vi "Status to Cluster.vi"(11 "Status":string) -> (3 "Status Cluster":T1)   [LabVIEW 2021, in "Keysight U1282A.lvlib"]
doc: "Este VI regresa la interpretación del status del instrumento (cadena de carácteres) en forma de un cluster de indicadores."
uses:
  Keysight U1282A.lvlib
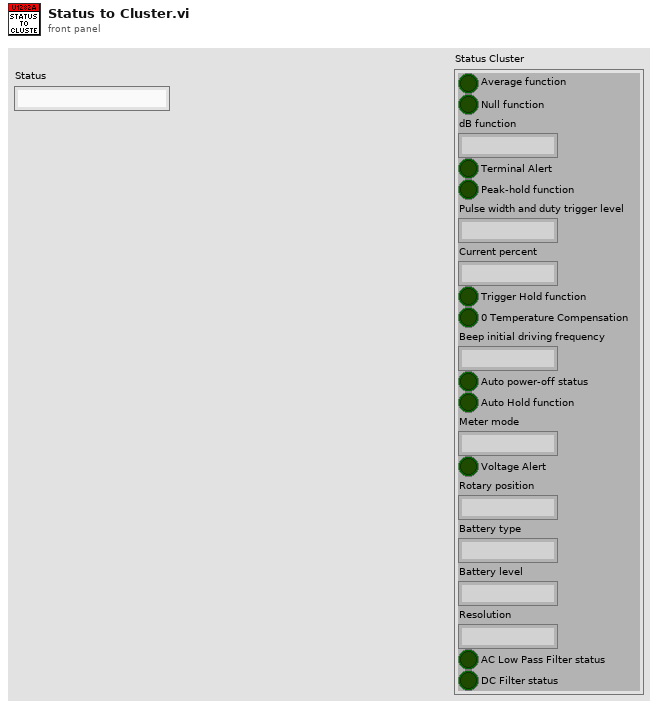
[diagram p1: front panel]
types:
  T1 = cluster{"Average function":bool, "Null function":bool, "dB function":string, "Terminal Alert":bool, "Peak-hold function":bool, "Pulse width and duty trigger level":string, "Current percent ":string, "Trigger Hold function":bool, "0 Temperature Compensation":bool, "Beep initial driving frequency":string, "Auto power-off status":bool, "Auto Hold function":bool, "Meter mode":string, "Voltage Alert":bool, "Rotary position":string, "Battery type":string, "Battery level":string, "Resolution":string, "AC Low Pass Filter status":bool, "DC Filter status":bool}
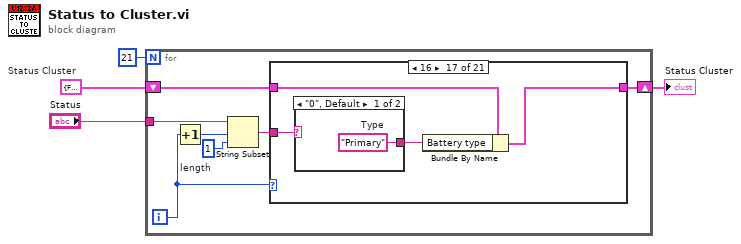
[diagram p0: block diagram]
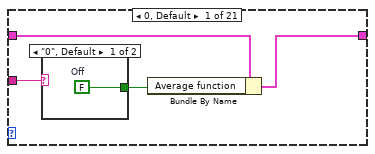
[diagram p2: hidden frame]
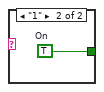
[diagram p3: hidden frame]
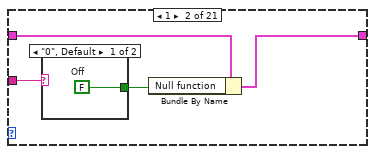
[diagram p4: hidden frame]
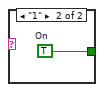
[diagram p5: hidden frame]
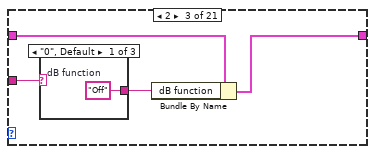
[diagram p6: hidden frame]
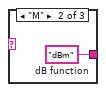
[diagram p7: hidden frame]
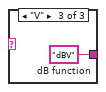
[diagram p8: hidden frame]
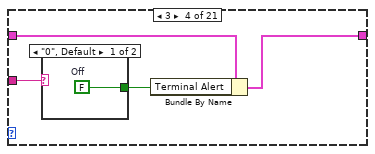
[diagram p9: hidden frame]
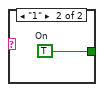
[diagram p10: hidden frame]
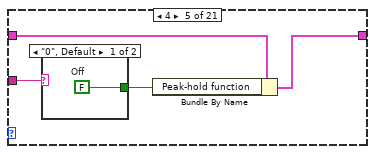
[diagram p11: hidden frame]
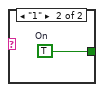
[diagram p12: hidden frame]
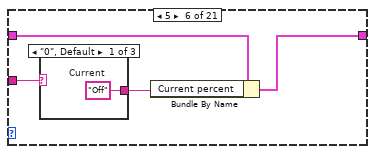
[diagram p13: hidden frame]
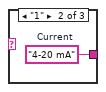
[diagram p14: hidden frame]
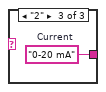
[diagram p15: hidden frame]
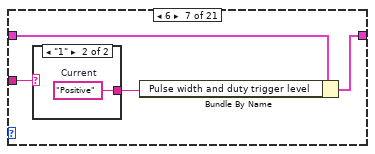
[diagram p16: hidden frame]
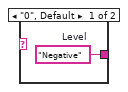
[diagram p17: hidden frame]
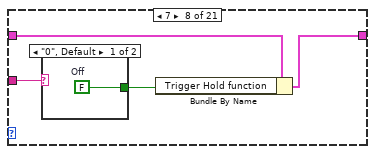
[diagram p18: hidden frame]
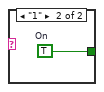
[diagram p19: hidden frame]
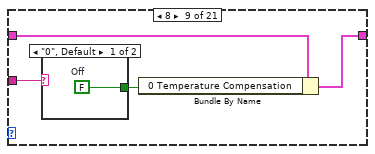
[diagram p20: hidden frame]
diagram:
  w1 = T1 {"Average function"=FALSE, "Null function"=FALSE, "dB function"="", "Terminal Alert"=FALSE, "Peak-hold function"=FALSE, "Pulse width and duty trigger level"="", "Current percent "="", "Trigger Hold function"=FALSE, "0 Temperature Compensation"=FALSE, "Beep initial driving frequency"="", "Auto power-off status"=FALSE, "Auto Hold function"=FALSE, "Meter mode"="", "Voltage Alert"=FALSE, "Rotary position"="", "Battery type"="", "Battery level"="", "Resolution"="", "AC Low Pass Filter status"=FALSE, "DC Filter status"=FALSE}  # Status Cluster
  n1 = for {
    N: 21 -> [_]
    tunnel: "Status" -> [w11]
    shift-right: [w8] -> w3
    shift-left: w1 -> [w9]
    i -> [w6]
    w10 = 1  # length
    n2 = Increment(x=w6) -> (x+1=w5:i32)
    n3 = String Subset(string=w11, offset (0)=w5, length (rest)=w10) -> (substring=w7:string)
    n4 = case shown="16" w6 {
      tunnel: w9 -> [w12 w18 w24 w34 w37 w43 w50 w56 w62 w68 w86 w95 w101 w107 w110 w111 w126 w134 w137 w143 w150]
      tunnel: [w13 w21 w27 w33 w40 w46 w53 w59 w65 w71 w89 w94 w100 w106 w110 w114 w125 w133 w140 w146 w149] -> w8
      tunnel: w7 -> [w15 w20 w26 w32 w39 w45 w52 w58 w64 w70 w88 w93 w99 w105 _ w113 w128 w132 w139 w145 w152]
      frame 0, Default {
        n5 = case shown="\"0\", Default" w15 {
          tunnel: [w16 w17] -> w14
          frame "0", Default {
            w16 = FALSE  # Off
          }
          frame "1" {
            w17 = TRUE  # On
          }
        }
        n6 = Bundle By Name(cluster=w12, "Average function"=w14) -> (w13:T1)
      }
      frame 1 {
        n7 = case shown="\"0\", Default" w20 {
          tunnel: [w22 w23] -> w19
          frame "0", Default {
            w22 = FALSE  # Off
          }
          frame "1" {
            w23 = TRUE  # On
          }
        }
        n8 = Bundle By Name(cluster=w18, "Null function"=w19) -> (w21:T1)
      }
      frame 2 {
        n9 = case shown="\"0\", Default" w26 {
          tunnel: [w28 w29 w30] -> w25
          frame "0", Default {
            w28 = "Off"  # dB function
          }
          frame "M" {
            w29 = "dBm"  # dB function
          }
          frame "V" {
            w30 = "dBV"  # dB function
          }
        }
        n10 = Bundle By Name(cluster=w24, "dB function"=w25) -> (w27:T1)
      }
      frame 3 {
        n11 = case shown="\"0\", Default" w32 {
          tunnel: [w35 w36] -> w31
          frame "0", Default {
            w35 = FALSE  # Off
          }
          frame "1" {
            w36 = TRUE  # On
          }
        }
        n12 = Bundle By Name(cluster=w34, "Terminal Alert"=w31) -> (w33:T1)
      }
      frame 4 {
        n13 = case shown="\"0\", Default" w39 {
          tunnel: [w41 w42] -> w38
          frame "0", Default {
            w41 = FALSE  # Off
          }
          frame "1" {
            w42 = TRUE  # On
          }
        }
        n14 = Bundle By Name(cluster=w37, "Peak-hold function"=w38) -> (w40:T1)
      }
      frame 5 {
        n15 = case shown="\"0\", Default" w45 {
          tunnel: [w47 w48 w49] -> w44
          frame "0", Default {
            w47 = "Off"  # Current
          }
          frame "1" {
            w48 = "4-20 mA"  # Current
          }
          frame "2" {
            w49 = "0-20 mA"  # Current
          }
        }
        n16 = Bundle By Name(cluster=w43, "Current percent"=w44) -> (w46:T1)
      }
      frame 6 {
        n17 = case shown="\"1\"" w52 {
          tunnel: [w54 w55] -> w51
          frame "0", Default {
            w54 = "Negative"  # Level
          }
          frame "1" {
            w55 = "Positive"  # Current
          }
        }
        n18 = Bundle By Name(cluster=w50, "Pulse width and duty trigger level"=w51) -> (w53:T1)
      }
      frame 7 {
        n19 = case shown="\"0\", Default" w58 {
          tunnel: [w60 w61] -> w57
          frame "0", Default {
            w60 = FALSE  # Off
          }
          frame "1" {
            w61 = TRUE  # On
          }
        }
        n20 = Bundle By Name(cluster=w56, "Trigger Hold function"=w57) -> (w59:T1)
      }
      frame 8 {
        n21 = case shown="\"0\", Default" w64 {
          tunnel: [w66 w67] -> w63
          frame "0", Default {
            w66 = FALSE  # Off
          }
          frame "1" {
            w67 = TRUE  # On
          }
        }
        n22 = Bundle By Name(cluster=w62, "0 Temperature Compensation"=w63) -> (w65:T1)
      }
      frame 9 {
        n23 = case shown="\"9\"" w70 {
          tunnel: [w72 w73 w74 w75 w76 w77 w78 w79 w80 w81 w82 w83 w84 w85] -> w69
          frame "0", Default {
            w72 = "Off"  # Frequency
          }
          frame "1" {
            w73 = "3200 Hz"  # Frequency
          }
          frame "2" {
            w74 = "3268 Hz"  # Frequency
          }
          frame "3" {
            w75 = "3339 Hz"  # Frequency
          }
          frame "4" {
            w76 = "3413 Hz"  # Frequency
          }
          frame "5" {
            w77 = "3491 Hz"  # Frequency
          }
          frame "6" {
            w78 = "3572 Hz"  # Frequency
          }
          frame "7" {
            w79 = "3657 Hz"  # Frequency
          }
          frame "8" {
            w80 = "3746 Hz"  # Frequency
          }
          frame "9" {
            w81 = "3840 Hz"  # Frequency
          }
          frame "A" {
            w82 = "3938 Hz"  # Frequency
          }
          frame "B" {
            w83 = "4042 Hz"  # Frequency
          }
          frame "C" {
            w84 = "4151 Hz"  # Frequency
          }
          frame "D" {
            w85 = "4267 Hz"  # Frequency
          }
        }
        n24 = Bundle By Name(cluster=w68, "Beep initial driving frequency"=w69) -> (w71:T1)
      }
      frame 10 {
        n25 = case shown="\"1\"" w88 {
          tunnel: [w90 w91] -> w87
          frame "0", Default {
            w90 = FALSE  # Off
          }
          frame "1" {
            w91 = TRUE  # On
          }
        }
        n26 = Bundle By Name(cluster=w86, "Auto power-off status"=w87) -> (w89:T1)
      }
      frame 11 {
        n27 = case shown="\"0\", Default" w93 {
          tunnel: [w96 w97] -> w92
          frame "0", Default {
            w96 = FALSE  # Off
          }
          frame "1" {
            w97 = TRUE  # On
          }
        }
        n28 = Bundle By Name(cluster=w95, "Auto Hold function"=w92) -> (w94:T1)
      }
      frame 12 {
        n29 = case shown="\"L\", Default" w99 {
          tunnel: [w102 w103] -> w98
          frame "L", Default {
            w102 = "Normal"  # Mode
          }
          frame "C" {
            w103 = "Calibraition"  # Mode
          }
        }
        n30 = Bundle By Name(cluster=w101, "Meter mode"=w98) -> (w100:T1)
      }
      frame 13 {
        n31 = case shown="\"0\", Default" w105 {
          tunnel: [w108 w109] -> w104
          frame "0", Default {
            w108 = FALSE  # Off
          }
          frame "1" {
            w109 = TRUE  # On
          }
        }
        n32 = Bundle By Name(cluster=w107, "Voltage Alert"=w104) -> (w106:T1)
      }
      frame 14 {
      }
      frame 15 {
        n33 = case shown="\"2\"" w113 {
          tunnel: [w115 w116 w117 w118 w119 w120 w121 w122 w123 w124] -> w112
          frame "0", Default {
            w115 = "ACV"  # Measurement
          }
          frame "1" {
            w116 = "ACmV"  # Measurement
          }
          frame "2" {
            w117 = "ACDCV"  # Measurement
          }
          frame "3" {
            w118 = "ACDCmV"  # Measurement
          }
          frame "4" {
            w119 = "Ohm/nS"  # Measurement
          }
          frame "5" {
            w120 = "Diode"  # Measurement
          }
          frame "6" {
            w121 = "CAP/Temp"  # Measurement
          }
          frame "7" {
            w122 = "uA/mA"  # Measurement
          }
          frame "8" {
            w123 = "Current"  # Measurement
          }
          frame "9" {
            w124 = "SQU"  # Measurement
          }
        }
        n34 = Bundle By Name(cluster=w111, "Rotary position"=w112) -> (w114:T1)
      }
      frame 16 {
        n35 = case shown="\"0\", Default" w128 {
          tunnel: [w129 w130] -> w127
          frame "0", Default {
            w129 = "Primary"  # Type
          }
          frame "1" {
            w130 = "Secondary"  # Type
          }
        }
        n36 = Bundle By Name(cluster=w126, "Battery type"=w127) -> (w125:T1)
      }
      frame 17 {
        n37 = case shown="\"0\", Default" w132 {
          tunnel: [w135 w136] -> w131
          frame "0", Default {
            w135 = "Normal"  # Level
          }
          frame "1" {
            w136 = "Low"  # Level
          }
        }
        n38 = Bundle By Name(cluster=w134, "Battery level"=w131) -> (w133:T1)
      }
      frame 18 {
        n39 = case shown="\"0\", Default" w139 {
          tunnel: [w141 w142] -> w138
          frame "0", Default {
            w141 = "Five decimals"  # Decimals
          }
          frame "1" {
            w142 = "Four Decimals"  # Decimals
          }
        }
        n40 = Bundle By Name(cluster=w137, "Resolution"=w138) -> (w140:T1)
      }
      frame 19 {
        n41 = case shown="\"0\", Default" w145 {
          tunnel: [w147 w148] -> w144
          frame "0", Default {
            w147 = FALSE  # Off
          }
          frame "1" {
            w148 = TRUE  # On
          }
        }
        n42 = Bundle By Name(cluster=w143, "AC Low Pass Filter status"=w144) -> (w146:T1)
      }
      frame 20 {
        n43 = case shown="\"0\", Default" w152 {
          tunnel: [w153 w154] -> w151
          frame "0", Default {
            w153 = FALSE  # Off
          }
          frame "1" {
            w154 = TRUE  # On
          }
        }
        n44 = Bundle By Name(cluster=w150, "DC Filter status"=w151) -> (w149:T1)
      }
    }
  }
  "Status Cluster" <- w3
